vi "Grep Strings.vi"(8 "match pattern":string, 11 "strings in":T1) -> (3 "strings out":T1)   [LabVIEW 2023]
uses:
  <extravilib>/ChannelInstances/Stream-str/)Channel.ctl
  <extravilib>/ChannelInstances/Stream-str/Read With Abort.vi
  <extravilib>/ChannelInstances/Stream-str/Write With Abort.vi
  <extravilib>/ChannelInstances/Stream-str/EndpointRead.vi
  <extravilib>/ChannelInstances/Stream-str/Endpoint.vi
  <extravilib>/ChannelInstances/Stream-str/)Channel.vi
  <resource>/ChannelSupport/_ChannelSupport/WaitIfNeeded.vi
  <extravilib>/ChannelInstances/Stream-str.lvlib
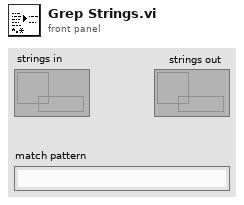
[diagram p1: front panel]
types:
  T1 = typedef "Stream-str.lvlib/)Channel.ctl" = refnum<queue>
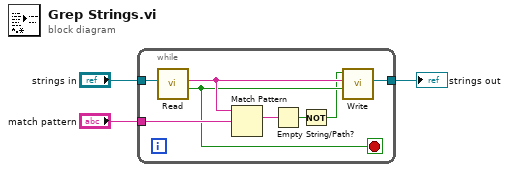
[diagram p0: block diagram]
diagram:
  n1 = while {
    tunnel: [w7] -> w3
    tunnel: "strings in" -> [w9]
    tunnel: "match pattern" -> [w11]
    stop <- w6 stop-if-true
    n2 = call <extravilib>:"Read.vi"("channel"=w9) -> ("last element?"=w6:bool, "element"=w8:string)  [unwired: 6 in, 3 out]
    n3 = Match Pattern(string=w8, regular expression=w11) -> (match substring=w10:string)  [unwired: 1 in, 3 out]
    n4 = Empty String/Path?(string/path=w10) -> (empty?=w5:bool)
    n5 = Not(x=w5) -> (.not. x?=w4:bool)
    n6 = call <extravilib>:"Write.vi"("last element? (F)"=w6, "element"=w8, "element valid? (T)"=w4) -> ("channel"=w7:T1)  [unwired: 6 in, 2 out]
  }
  "strings out" <- w3
